vi "testLaserComms.vi"() -> ()   [LabVIEW 2015]
panel:
  out "x/y":dbl
  out "read buffer":string
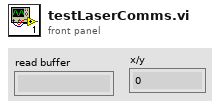
[diagram p1: front panel]
types:
  T1 = cluster{"Device Name":string, "Firmware":string, "S/N":string, "Firmware Head":string, "S/N Head":string, "Wavelength":string, "Spec Power":string}
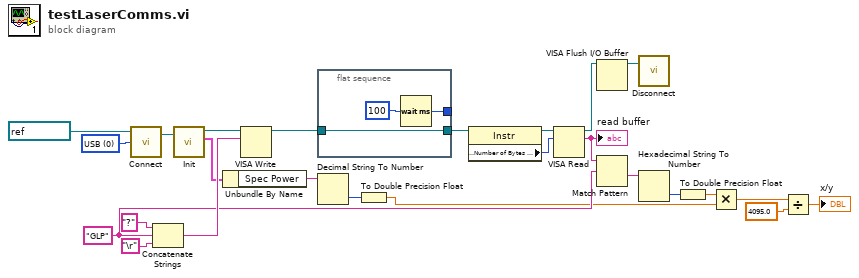
[diagram p0: block diagram]
diagram:
  w11 = "GLP" ("Schreibpuffer")
  w24 = u16 0 items=["USB", "RS232"] ("Connection type")
  n1 = call "Connect.vi"("Connection type"=w24, "Com Port"=refnum<visa-resource-name> "COM4") -> ("VISA resource name out"=w23:refnum<visa-resource-name>)  [unwired: 1 in, 1 out]
  n2 = Concatenate Strings("?" ("string"), w11, "\r") -> (w21:string)
  n3 = call "Init.vi"("Com Port in"=w23) -> ("COM Port out"=w20:refnum<visa-resource-name>, "Device Information"=w9:T1)  [unwired: 1 in, 2 out]
  n4 = Unbundle By Name(w9) -> ("Spec Power"=w8:string)
  n5 = VISA Write(VISA resource name=w20, write buffer=w21) -> (VISA resource name out=w19:refnum<visa-resource-name>)  [unwired: 1 in, 2 out]
  n6 = flat-sequence {
    tunnel: w19 -> [w28]
    tunnel: [w28] -> w18
    tunnel: [w26] -> _
    frame #0 {
      n7 = Wait (ms)(milliseconds to wait=u32 100) -> (millisecond timer value=w26:u32)
    }
  }
  n8 = Decimal String To Number(string=w8) -> (number=w4:i32)  [unwired: 2 in, 1 out]
  n9 = To Double Precision Float(number=w4) -> (double precision float=w5:dbl)
  n10 = property class="Instr"(reference=w18) -> (reference out=w17:refnum<visa-resource-name>, "Serial Settings:Number of Bytes at Serial Port"=w16:u32)  [unwired: 1 in, 1 out]
  n11 = VISA Read(VISA resource name=w17, byte count=w16) -> (VISA resource name out=w15:refnum<visa-resource-name>, read buffer=w13:string)  [unwired: 1 in, 2 out]
  "read buffer" <- w13
  n12 = VISA Flush I/O Buffer(VISA resource name=w15) -> (VISA resource name out=w14:refnum<visa-resource-name>)  [unwired: 2 in, 1 out]
  n13 = Match Pattern(string=w13, regular expression=w11) -> (after substring=w10:string)  [unwired: 1 in, 3 out]
  n14 = call "Disconnect.vi"("Com Port in"=w14) -> ()  [unwired: 1 in, 1 out]
  n15 = Hexadecimal String To Number(string=w10) -> (number=w7:u32)  [unwired: 2 in, 1 out]
  n16 = To Double Precision Float(number=w7) -> (double precision float=w6:dbl)
  n17 = Multiply(x=w6, y=w5) -> (x*y=w3:dbl)
  n18 = Divide(x=w3, y=4095.0) -> (x/y=→"x/y":dbl)
